vi "NIIE_Analyze XML stream.vi"(11 "XML Data":T1[](array[typedef])) -> (3 "Data":T2(array[cluster]))   [LabVIEW 2021]
uses:
  Controls/XMLDataStructureIconLibrary.ctl
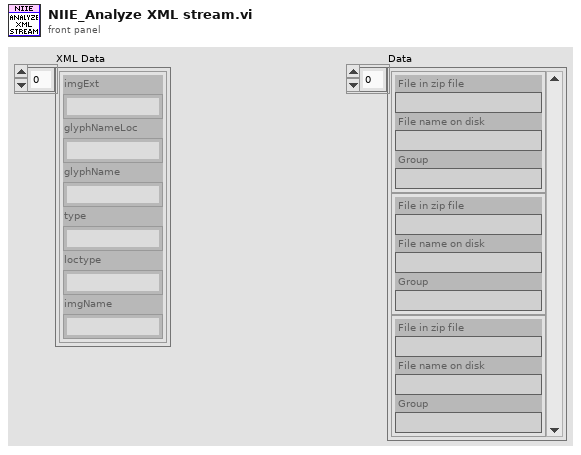
[diagram p1: front panel]
types:
  T1 = typedef "XMLDataStructureIconLibrary.ctl" = cluster{"imgExt":string, "glyphNameLoc":string, "glyphName":string, "type":string, "loctype":string, "imgName":string}
  T2 = cluster{"File in zip file":string, "File name on disk":string, "Group":string}[]
  T3 = cluster{"File name in zip file":string, "File name on disk":string, "Group":string}
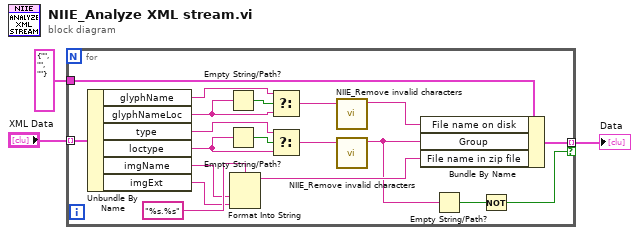
[diagram p0: block diagram]
diagram:
  n1 = for {
    tunnel: [w22] -> w3 mode=indexing if=w4
    tunnel: "XML Data" -> [w16] mode=indexing
    tunnel: T3 {"File name in zip file"="", "File name on disk"="", "Group"=""} ("cluster") -> [w18]
    n2 = Unbundle By Name(w16) -> ("glyphName"=w15:string, "glyphNameLoc"=w14:string, "type"=w13:string, "loctype"=w12:string, "imgName"=w11:string, "imgExt"=w10:string)
    n3 = Empty String/Path?(string/path=w14) -> (empty?=w21:bool)
    n4 = Empty String/Path?(string/path=w12) -> (empty?=w20:bool)
    n5 = Format Into String(format string="%s.%s", w11, w10) -> (resulting string=w17:string)  [unwired: 2 in, 1 out]
    n6 = Select(t=w15, s=w21, f=w14) -> (s? t:f=w8:string)
    n7 = Select(t=w13, s=w20, f=w12) -> (s? t:f=w9:string)
    n8 = call "NIIE_Remove invalid characters.vi"("String in"=w8) -> ("Filtered string out"=w7:string)  [unwired: 10 in]
    n9 = call "NIIE_Remove invalid characters.vi"("String in"=w9) -> ("Filtered string out"=w6:string)  [unwired: 10 in]
    n10 = Bundle By Name(cluster=w18, "File name on disk"=w7, "Group"=w6, "File name in zip file"=w17) -> (w22:T3)
    n11 = Empty String/Path?(string/path=w6) -> (empty?=w5:bool)
    n12 = Not(x=w5) -> (.not. x?=w4:bool)
  }
  "Data" <- w3
